vi "Send Set Stage Speed.vi"(7 "Message Priority (Normal)":T1=enum."Normal", 8 "error in (no error)":errorcluster, 9 "Y Axis":u16, 10 "X Axis":u16, 11 "Interlock Q Class in":refnum<class "Interlock Q Class.lvclass">) -> (0 "error out":errorcluster, 3 "Interlock Q Class out":refnum<class "Interlock Q Class.lvclass">)   [LabVIEW 2022 SP3, in "XY Stage Process.lvlib" / "Set Stage Speed Msg.lvclass"]
doc: "This VI sends the message to an actor."
uses:
  Set Stage Speed Msg.lvclass
  Set Stage Speed Msg.lvclass/Set Stage Speed Msg.ctl
  Process Framework/Interlock Q Class/Interlock Q Class.lvclass
  <vilib>/ActorFramework/Message Enqueuer/Message Priority.ctl
  <vilib>/ActorFramework/Message Enqueuer/Message Enqueuer.lvclass
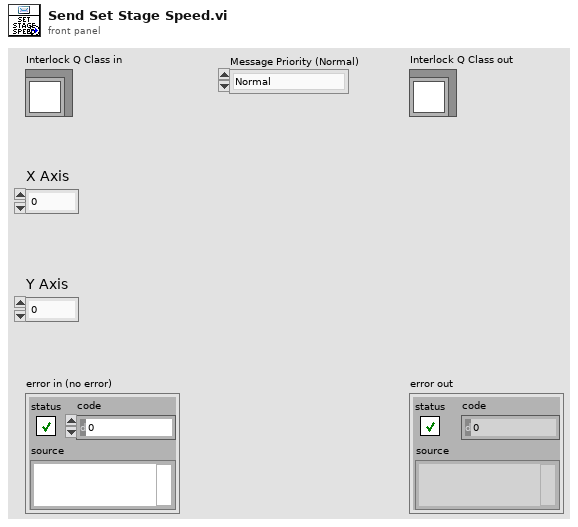
[diagram p1: front panel]
types:
  T1 = typedef "Actor Framework.lvlib/Message Enqueuer.lvclass/Message Priority.ctl" = enum16{"Low", "Normal", "High"}
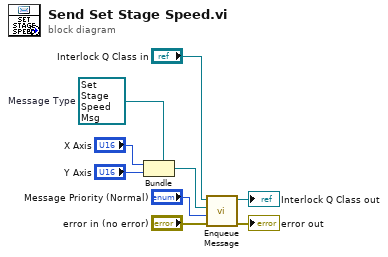
[diagram p0: block diagram]
diagram:
  w9 = refnum<class "Set Stage Speed Msg.lvclass"> refnum  # Message Type
  n1 = Bundle(cluster=w9, "X Axis", "Y Axis") -> (w4:refnum<class "Set Stage Speed Msg.lvclass">)
  n2 = call-dynamic "Enqueue Message.vi"("error in (no error)"="error in (no error)", "Message Priority (Normal)"="Message Priority (Normal)", "Message"=w4, "Interlock Q Class in"="Interlock Q Class in") -> ("error out"=→"error out":errorcluster, "Interlock Q Class out"=→"Interlock Q Class out":refnum<class "Interlock Q Class.lvclass">)  [unwired: 6 in]
